vi "Lookup Service.vi"(7 "Service Type / ID":refnum<class "Service.lvclass">, 8 "error in (no error)":errorcluster, 11 "Vecto in":refnum<class "Vecto.lvclass">) -> (0 "error out":errorcluster, 2 "Service":refnum<class "Service.lvclass">, 3 "Vecto out":refnum<class "Vecto.lvclass">)   [LabVIEW 2020, in "Vecto.lvlib" / "Vecto.lvclass"]
uses:
  Vecto.lvclass
  Service/Service.lvclass
  Vecto.lvclass/Vecto.ctl
  Service Container/Service Container.lvclass
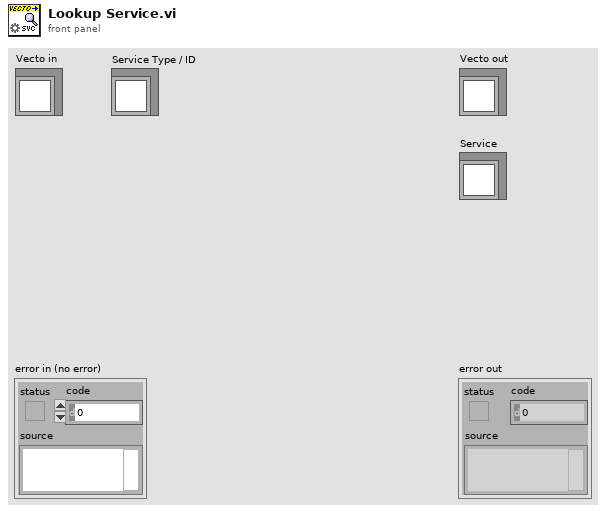
[diagram p1: front panel]
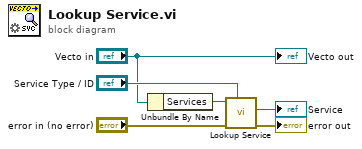
[diagram p0: block diagram]
diagram:
  n1 = Unbundle By Name("Vecto in") -> ("Services"=w6:refnum<class "Service Container.lvclass">)
  n2 = call "Lookup Service.vi"("Service Lookup"="Service Type / ID", "error in (no error)"="error in (no error)", "Service Container in"=w6) -> ("error out"=→"error out":errorcluster, "Service"=→"Service":refnum<class "Service.lvclass">)  [unwired: 6 in, 1 out]
  "Vecto out" <- "Vecto in"
